vi "Get Rotation.vi"(8 "error in (no error)":errorcluster, 11 "Scene Object":refnum<vi>) -> (0 "error out":errorcluster, 1 "Angle":sgl, 2 "Axis":cluster{"X":sgl, "Y":sgl, "Z":sgl}, 3 "Scene Object":refnum<vi>)   [LabVIEW 2017, in "NI_3D Picture Control.lvlib"]
doc: "Returns the rotation applied to an object in a 3D scene in axis-angle form."
uses:
  <vilib>/picture/3D Picture Control/NI_3D Picture Control.lvlib
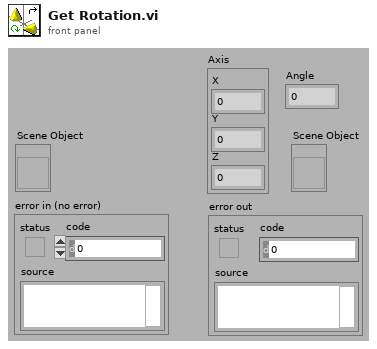
[diagram p1: front panel]
types:
  T1 = typedef "LV3DPointTypeDef.ctl" = cluster{"X":sgl, "Y":sgl, "Z":sgl}
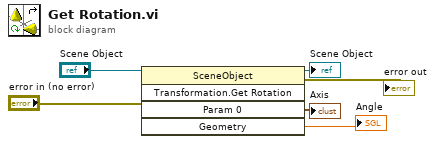
[diagram p0: block diagram]
diagram:
  n1 = invoke class="SceneObject" method="Transformation.Get Rotation"(reference="Scene Object", error in="error in (no error)") -> (reference out=→"Scene Object":refnum<vi>, error out=→"error out":errorcluster, "Param 0"=→"Axis":T1, "Geometry"=→"Angle":sgl)  [unwired: 3 in, 1 out]
